vi "main.vi"() -> ()   [LabVIEW 2019]
uses:
  <vilib>/addons/database/Auxilliary.llb/DB Tools Column Info.ctl
  <vilib>/addons/database/Auxilliary.llb/DB Tools DataTypes.ctl
  <vilib>/addons/database/NI_Database_API.lvlib
panel:
  out "error out 2":errorcluster
  in  "column information":T1[](array[typedef])
  in  "?":bool
  out "data":cluster{string, i32, dbl}[](array[cluster])
  out "error out":errorcluster
  in  "value_in_the_field_to_find":string
  in  "select_the_field_to_search":string(combo)
  in  "stop":bool
  in  "OK Button":bool
  in  "Cluster":T3
  in  "table":string
  in  "connection information":path
  in  "Combo Box":string(combo)
  # "tabble_creation"
  # "inserting_data"
  # "finding_value"
  # "enter the new table name in above table box"
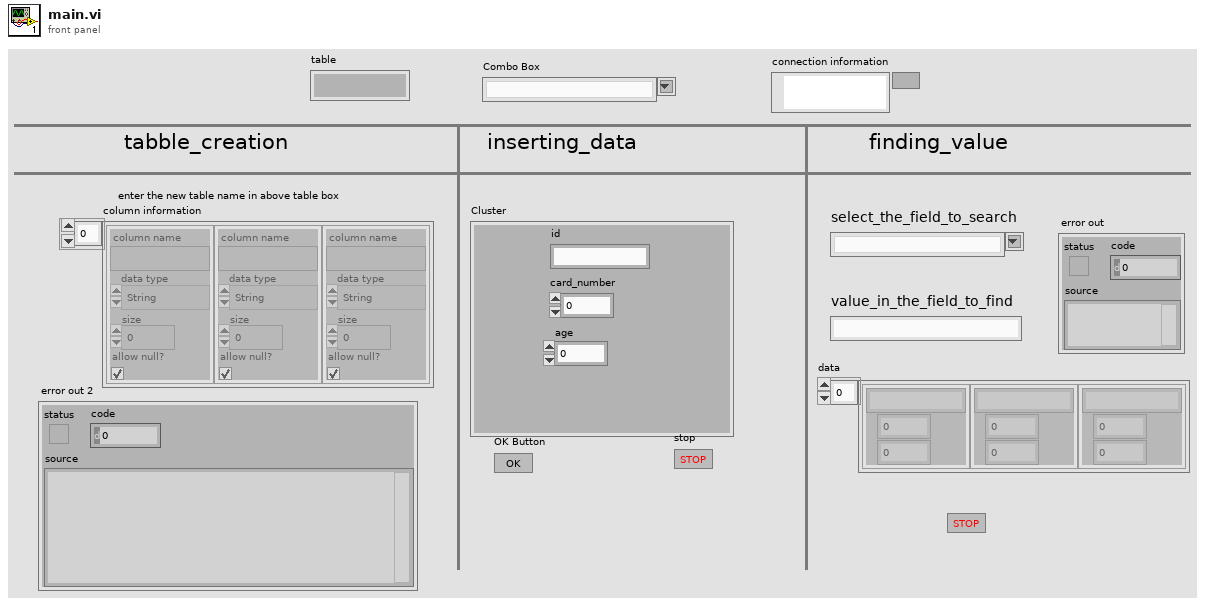
[diagram p1: front panel]
types:
  T1 = typedef "NI_Database_API.lvlib/DB Tools Column Info.ctl" = cluster{"column name":string, "data type":T2, "size":i32, "allow null?":bool}
  T2 = typedef "NI_Database_API.lvlib/DB Tools DataTypes.ctl" = enum16{"String", "Long (I32)", "Single (SGL)", "Double (DBL)", "Date/Time", "Binary"}
  T3 = cluster{"id":string, "card_number":dbl, "age":dbl}
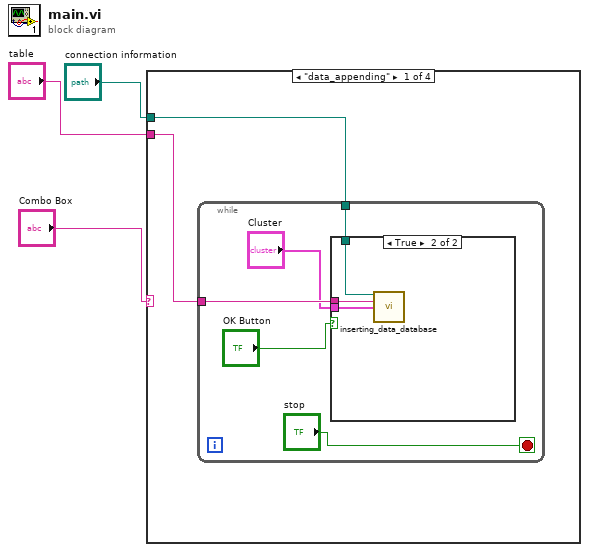
[diagram p0: block diagram]
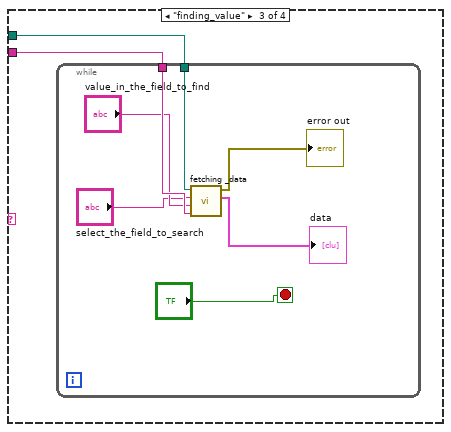
[diagram p4: hidden frame]
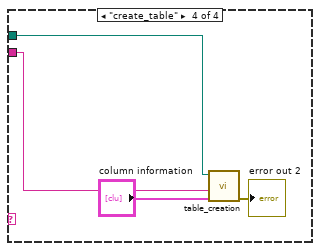
[diagram p5: hidden frame]
diagram:
  n1 = case shown="\"data_appending\"" "Combo Box" {
    tunnel: "connection information" -> [w5 _ w15 w26]
    tunnel: "table" -> [w4 _ w14 w25]
    frame "data_appending" {
      n2 = while {
        tunnel: w5 -> [w10]
        tunnel: w4 -> [w9]
        stop <- "stop" stop-if-true
        n3 = case shown="True" "OK Button" {
          tunnel: w10 -> [_ w13]
          tunnel: w9 -> [_ w12]
          tunnel: "Cluster" -> [_ w11]
          frame False {
          }
          frame True {
            n4 = call "inserting_data_database.vi"("connection information"=w13, "table"=w12, "Cluster"=w11) -> ()  [unwired: 13 in]
          }
        }
      }
    }
    frame Default {
    }
    frame "finding_value" {
      n5 = while {
        tunnel: w15 -> [w22]
        tunnel: w14 -> [w21]
        stop <- "?" stop-if-true
        n6 = call "fetching _data.vi"("table"=w21, "value_in_the_field_to_find"="value_in_the_field_to_find", "select_the_field_to_search"="select_the_field_to_search", "database_link"=w22) -> ("data"=→"data":cluster{string, i32, dbl}[], "error out"=→"error out":errorcluster)  [unwired: 6 in]
      }
    }
    frame "create_table" {
      n7 = call "table_creation.vi"("column information"="column information", "table_name"=w25, "connection information"=w26) -> ("error out"=→"error out 2":errorcluster)  [unwired: 8 in]
    }
  }
